vi "Finalize.vi"(8 "error in":errorcluster, 11 "logging execution unit":refnum<class "Logging Execution Unit.lvclass">) -> (0 "error out":errorcluster, 3 "logging execution unit out":refnum<class "Logging Execution Unit.lvclass">)   [LabVIEW 2020, in "AIM MIL-STD-1553 Engine.lvlib" / "Implementation.lvlib" / "Logging Execution Unit.lvclass"]
uses:
  Logging Execution Unit.lvclass
  C:/dev/git/niveristand-aim-milStd1553-custom-device/Source/Custom Device Support/Engine/Implementation/Execution Unit/Execution Unit.lvclass
  Execution Unit/Execution Unit.lvclass/Execution Unit.ctl
  Execution Unit/Execution Unit.lvclass
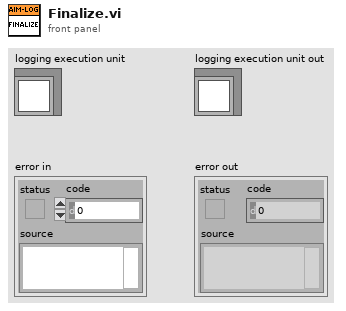
[diagram p1: front panel]
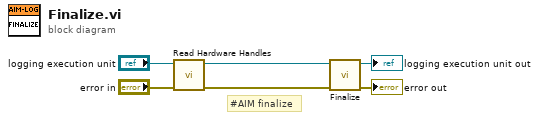
[diagram p0: block diagram]
diagram:
  # "#AIM finalize"
  n1 = call "Read Hardware Handles.vi"("error in"="error in", "Execution Unit in"="logging execution unit") -> ("error out"=w2:errorcluster, "Execution Unit out"=w1:refnum<class "Logging Execution Unit.lvclass">)  [unwired: 7 in, 1 out]
  n2 = call-parent "Finalize.vi"("error in (no error)"=w2, "Execution Unit Implementation in"=w1) -> ("error out"=→"error out":errorcluster, "Execution Unit Implementation out"=→"logging execution unit out":refnum<class "Logging Execution Unit.lvclass">)  [unwired: 8 in]
